vi "Initialize Strain Config.vi"   [LabVIEW 2019, in "GaitDAQ UI.lvlib"]
uses:
  GaitDAQ UI.lvlib
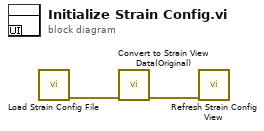
[diagram p0: block diagram]
diagram:
  n1 = call "Load Strain Config File.vi"() -> ("error out"=w2:errorcluster)  [unwired: 11 in]
  n2 = call "Convert to Strain View Data(Original).vi"("error in (no error)"=w2) -> ("error out"=w1:errorcluster)  [unwired: 10 in]
  n3 = call "Refresh Strain Config View.vi"("error in (no error)"=w1) -> ()  [unwired: 10 in, 1 out]
